vi "Increment Build Number.vi"(0 "NI Build Specification in":refnum<class "Installer_LV.lvclass">, 11 "error in (no error)":errorcluster) -> (4 "NI Build Specification out":refnum<class "Installer_LV.lvclass">, 15 "error out":errorcluster)   [LabVIEW 2017, in "CL_G3_VIComponentBuilder.lvlib" / "Installer_LV.lvclass"]
doc: "Increments the build number of the installer in the LabVIEW Project build spec."
uses:
  Installer_LV.lvclass
  C:/builds/Component BuilderBT/SrcDist/Exports/Exports/Export.lvclass
  C:/builds/Component BuilderBT/SrcDist/Exports/NI Build Specification_LV/NI Build Specification_LV.lvclass
  Exports/Export.lvclass/Export.ctl
  NI Build Specification_LV/NI Build Specification_LV.lvclass/NI Build Specification_LV.ctl
  Exports/Accessors/Read Exported Build Specification Path.vi
  NI Build Specification_LV/Accessors/Read Build Number XML Prop Name.vi
  <vilib>/xml/Load XML File.vi
  <vilib>/xml/Close Reference(Node).vi
  <vilib>/xml/NI_XML.lvlib
  <resource>/objmgr/DOMUserDefRef.rc
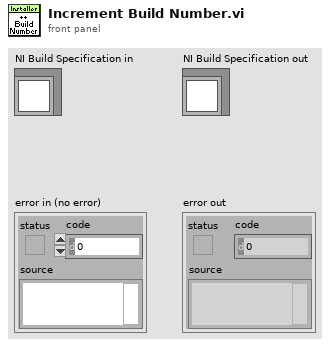
[diagram p1: front panel]
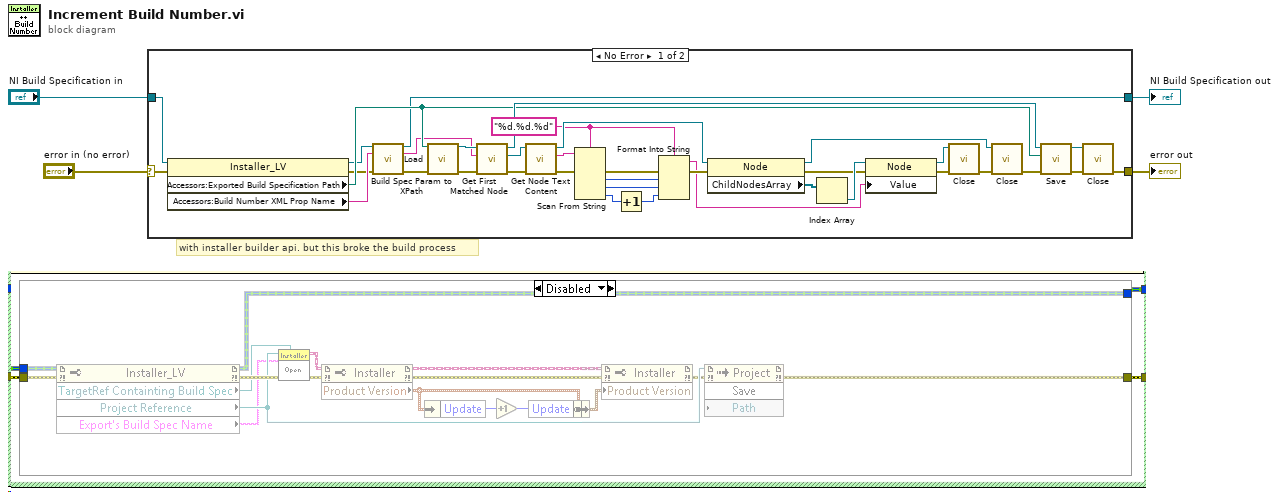
[diagram p0: block diagram]
diagram:
  # "with installer builder api. but this broke the build process"
  n1 = case shown="No Error" "error in (no error)" {
    selector: "error in (no error)" -> [w40 w41]
    tunnel: [w12 w41] -> w3
    tunnel: "NI Build Specification in" -> [w39 w42]
    tunnel: [w10 w42] -> w1
    frame No Error {
      w20 = "%d.%d.%d" ("format string")
      n2 = property class="Installer_LV"(reference=w39, error in=w40) -> (reference out=w11:refnum<class "Installer_LV.lvclass">, error out=w7:errorcluster, "Accessors:Exported Build Specification Path"=w22:path, "Accessors:Build Number XML Prop Name"=w9:string)
      n3 = call-dynamic "Build Spec Param to XPath.vi"("NI Build Specification"=w11, "Build Spec Parameter Name"=w9, "error in (no error)"=w7) -> ("NI Build Specification"=w10:refnum<class "Installer_LV.lvclass">, "XPath to the specific build Spec Property"=w8:string, "error out"=w6:errorcluster)  [unwired: 10 in]
      n4 = call-poly <vilib>:"Load.vi"("path to XML document"=w22, "error in (no error)"=w6) -> ("DOM document out"=w24:refnum<k20>, "error out"=w23:errorcluster)  [unwired: 11 in, 1 out]
      n5 = call <vilib>:"Get First Matched Node.vi"("error in (no error)"=w23, "XPath expression"=w8, "node in"=w24) -> ("error out"=w34:errorcluster, "node result"=w35:refnum<k20>, "node out"=w32:refnum<k20>)  [unwired: 6 in]
      n6 = call <vilib>:"Get Node Text Content.vi"("error in (no error)"=w34, "node in"=w35) -> ("error out"=w16:errorcluster, "node text"=w5:string, "node out"=w33:refnum<k20>)  [unwired: 7 in]
      n7 = Scan From String(format string=w20, input string=w5, error in=w16) -> (error out=w15:errorcluster, output 1=w19:i32, output 2=w18:i32, output 3=w21:i32)  [unwired: 4 in, 2 out]
      n8 = Increment(x=w21) -> (x+1=w17:i32)
      n9 = Format Into String(format string=w20, error in=w15, w19, w18, w17) -> (resulting string=w13:string, error out=w14:errorcluster)  [unwired: 1 in]
      n10 = property class="Node"(reference=w33, error in=w14) -> (reference out=w38:refnum<k20>, error out=w25:errorcluster, "ChildNodesArray"=w30:refnum<k20>[])
      n11 = Index Array(array=w30) -> (element=w29:refnum<k20>)  [unwired: 1 in]
      n12 = property class="Node"(reference=w29, error in=w25, "Value"=w13) -> (reference out=w27:refnum<k20>, error out=w28:errorcluster)
      n13 = call-poly <vilib>:"Close.vi"("error in (no error)"=w28, "node"=w27) -> ("error out"=w26:errorcluster)  [unwired: 7 out]
      n14 = call-poly <vilib>:"Close.vi"("error in (no error)"=w26, "node"=w38) -> ("error out"=w31:errorcluster)  [unwired: 7 in]
      n15 = call <vilib>:"Save.vi"("error in (no error)"=w31, "XML file path"=w22, "DOM document in"=w32) -> ("error out"=w36:errorcluster, "DOM document out"=w37:refnum<k20>)  [unwired: 6 in, 1 out]
      n16 = call-poly <vilib>:"Close.vi"("error in (no error)"=w36, "node"=w37) -> ("error out"=w12:errorcluster)  [unwired: 7 in]
    }
    frame Error {
    }
  }
  "error out" <- w3
  "NI Build Specification out" <- w1
